vi "Ultramat 23 AFCO Calculations.vi"(8 "error in (no error)":errorcluster, 9 "Measured variables":T1[](array[typedef]), 10 "Measurements":cluster{"Measured value":dbl, "Dimension":T2}[](array[cluster]), 11 "Gas selected":string) -> (0 "error out":errorcluster, 1 "Measured variables Output":T1[](array[typedef]), 2 "Measurements Output":cluster{"Measured value":dbl, "Dimension":T2}[](array[cluster]), 5 "AFCO Data":string[][](array[string]))   [LabVIEW 2023]
uses:
  instr.lib/Siemens ELAN/Measured variables.ctl
  instr.lib/Siemens ELAN/Unit Dimensions.ctl
  instr.lib/Siemens ELAN/Siemens ELAN.lvlib
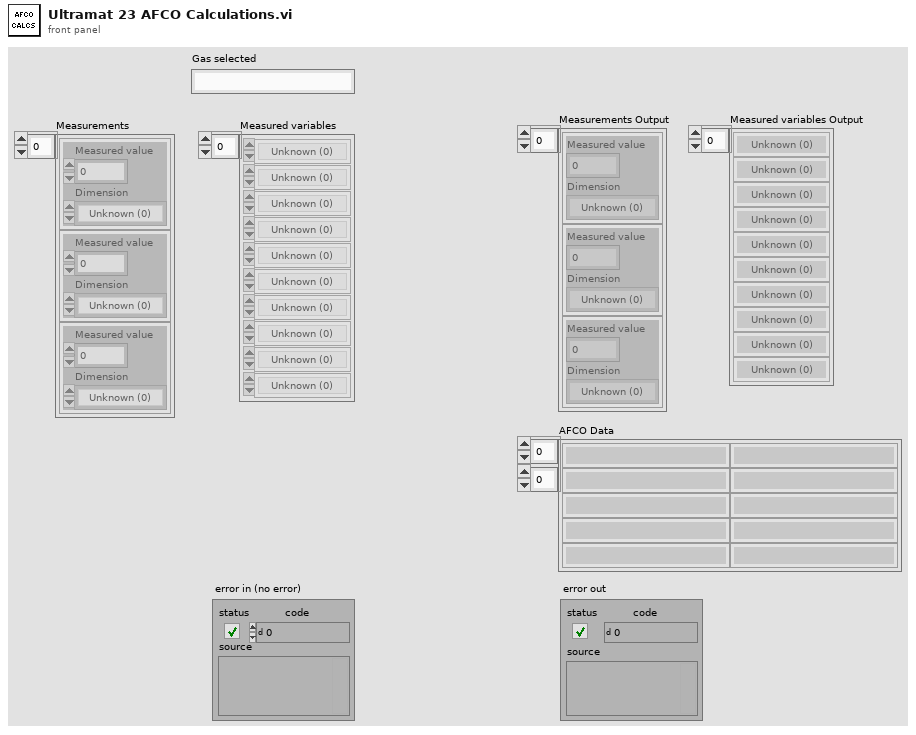
[diagram p1: front panel]
types:
  T1 = typedef "Siemens ELAN.lvlib/Measured variables.ctl" = enum8{"Unknown (0)", "No component", "CO", "CO2", "CH4", "C6H14", "SO2", "NO", "NO2", "CHClF2 (R22)", "C3H8", "C4H10", "O2", "C5H12", "HC", "Pressure", "pH", "Temperature", "C2H4", "C2H2", "C3H6", "C4H6", "C4H8", "C2H6", "NH3", "N2O", "C6H6", "SF6", "CH3OH", "C2H5OH", "CH2Cl2", "C2H4Cl2", "CH3Cl", "C2H4O", "H2O (vapor)", "G/l", "Unknown (36)", "Unknown (37)", "Unknown (38)", "Unknown (39)", "Unknown (40)", "Unknown (41)", "Unknown (42)", "Unknown (43)", "Unknown (44)", "Unknown (45)", "Unknown (46)", "Unknown (47)", "Unknown (48)", "Unknown (49)", "Unknown (50)", "Unknown (51)", "Unknown (52)", "Unknown (53)", "Unknown (54)", "Unknown (55)", "Unknown (56)", "Unknown (57)", "Unknown (58)", "Unknown (59)", "Unknown (60)", "Unknown (61)", "Unknown (62)", "Unknown (63)", "Unknown (64)", "Unknown (65)", "Unknown (66)", "Unknown (67)", "Unknown (68)", "Unknown (69)", "Unknown (70)", "Unknown (71)", "Unknown (72)", "Unknown (73)", "Unknown (74)", "Unknown (75)", "Unknown (76)", "Unknown (77)", "Unknown (78)", "Unknown (79)", "Unknown (80)", "Unknown (81)", "Unknown (82)", "Unknown (83)", "Unknown (84)", "Unknown (85)", "Unknown (86)", "Unknown (87)", "Unknown (88)", "Unknown (89)", "Unknown (90)", "Unknown (91)", "Unknown (92)", "Unknown (93)", "Unknown (94)", "Unknown (95)", "Unknown ((96)", "Unknown (97)", "Unknown (98)", "Unknown (99)", "Ambient Pressure", "Unknown (>100)"}
  T2 = typedef "Siemens ELAN.lvlib/Unit Dimensions.ctl" = enum8{"Unknown (0)", "Pure number", "ppm", "ppb", "vpm", "vpm C1", "vpm C3", "vpm C6", "mg C/m^3", "mg/m^3", "%", "% v/v", "% of range", "% saturation", "%/°C", "%/K", "% w/w", "mV/pH", "mV/mbar", "nA/mbar", "S/m", "S/cm", "mS/m", "mS/cm", "uS/m", "uS/cm", "s", "min", "hr", "pA", "mA", "uV", "mV", "V", "mbar", "hPa", "ml/min", "kohm", "MOhm", "S", "°C", "Hz", "pH", "ug/l", "mg/l", "l/min", "uA", "mg/dm^3", "kPa", "kohm*cm", "MOhm*cm", "°", "Unknown (>51)"}
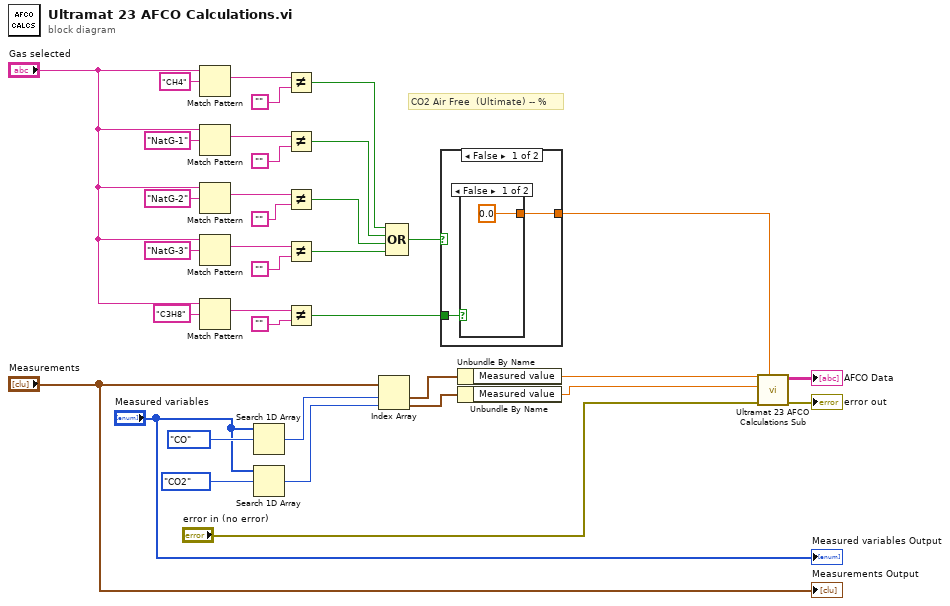
[diagram p0: block diagram]
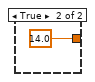
[diagram p2: hidden frame]
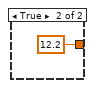
[diagram p3: hidden frame]
diagram:
  # "CO2 Air Free  (Ultimate) -- %"
  n1 = Match Pattern(string="Gas selected", regular expression="CH4") -> (match substring=w26:string)  [unwired: 1 in, 3 out]
  n2 = Match Pattern(string="Gas selected", regular expression="NatG-1") -> (match substring=w8:string)  [unwired: 1 in, 3 out]
  n3 = Match Pattern(string="Gas selected", regular expression="NatG-2") -> (match substring=w5:string)  [unwired: 1 in, 3 out]
  n4 = Match Pattern(string="Gas selected", regular expression="NatG-3") -> (match substring=w27:string)  [unwired: 1 in, 3 out]
  n5 = Match Pattern(string="Gas selected", regular expression="C3H8") -> (match substring=w34:string)  [unwired: 1 in, 3 out]
  n6 = Search 1D Array(1D array="Measured variables", element=Measured_variables."CO" ("Measured variable")) -> (index of element=w21:i32)  [unwired: 1 in]
  n7 = Search 1D Array(1D array="Measured variables", element=Measured_variables."CO2" ("Measured variable")) -> (index of element=w20:i32)  [unwired: 1 in]
  n8 = Not Equal?(x=w26, y="") -> (x != y?=w30:bool)
  n9 = Not Equal?(x=w8, y="") -> (x != y?=w2:bool)
  n10 = Not Equal?(x=w5, y="") -> (x != y?=w1:bool)
  n11 = Not Equal?(x=w27, y="") -> (x != y?=w31:bool)
  n12 = Not Equal?(x=w34, y="") -> (x != y?=w36:bool)
  n13 = Index Array(array="Measurements", index #1=w21, index #2=w20) -> (element #1=w17:cluster{"Measured value":dbl, "Dimension":T2}, element #2=w16:cluster{"Measured value":dbl, "Dimension":T2})
  n14 = Compound Arithmetic op=OR(w30, w2, w1, w31) -> (w35:bool)
  n15 = case shown="False" w35 {
    tunnel: w36 -> [w38 _]
    tunnel: [w37 12.2] -> w14
    frame False {
      n16 = case shown="False" w38 {
        tunnel: [0.0 14.0] -> w37
        frame False {
        }
        frame True {
        }
      }
    }
    frame True {
    }
  }
  n17 = Unbundle By Name(w17) -> ("Measured value"=w13:dbl)
  n18 = Unbundle By Name(w16) -> ("Measured value"=w12:dbl)
  n19 = call "Ultramat 23 AFCO Calculations Sub.vi"("CO2 Air Free-Ultimate (%)"=w14, "error in (no error)"="error in (no error)", "CO2 (%)"=w12, "CO (PPMv)"=w13) -> ("error out"=→"error out":errorcluster, "AFCO Data"=→"AFCO Data":string[][])  [unwired: 6 in]
  "Measurements Output" <- "Measurements"
  "Measured variables Output" <- "Measured variables"
